vi "Q_learning_get_env_feedback.vi"(8 "A":string, 10 "S":string) -> (0 "R":dbl, 2 "S_":string)   [LabVIEW 2010]
uses:
  Q_learning_Global.vi
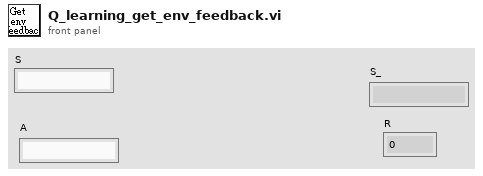
[diagram p1: front panel]
types:
  T1 = cluster{"N_STATES":dbl, "EPSILON":dbl, "ALPHA":dbl, "GAMMA":dbl, "MAX_EPISODES":dbl, "FRESH_TIME":dbl, "ACTIONS":string[]}
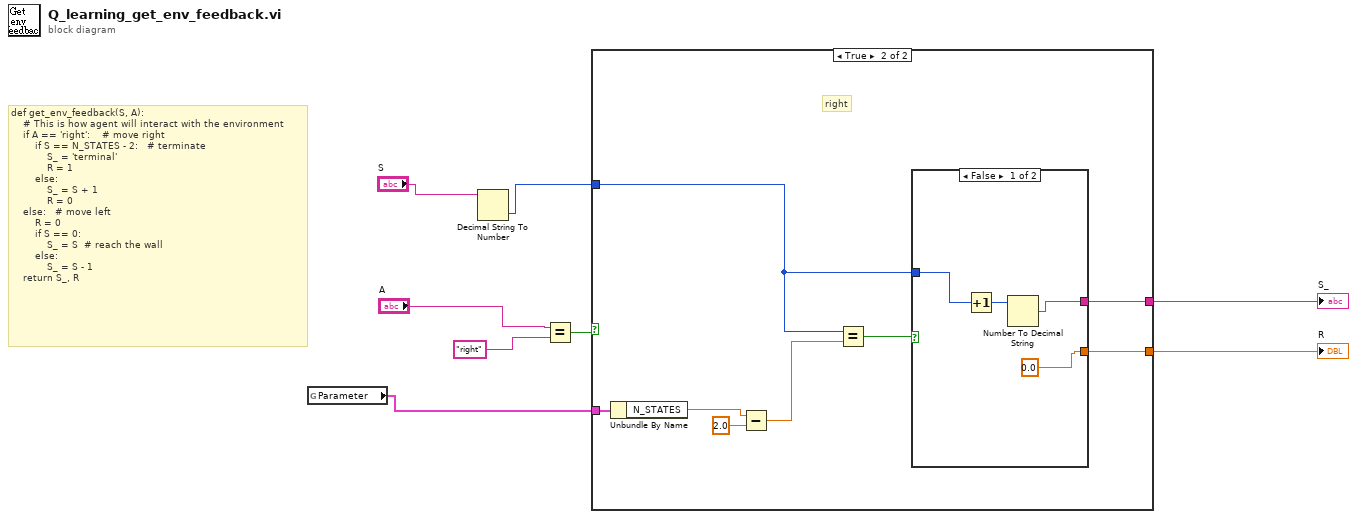
[diagram p0: block diagram]
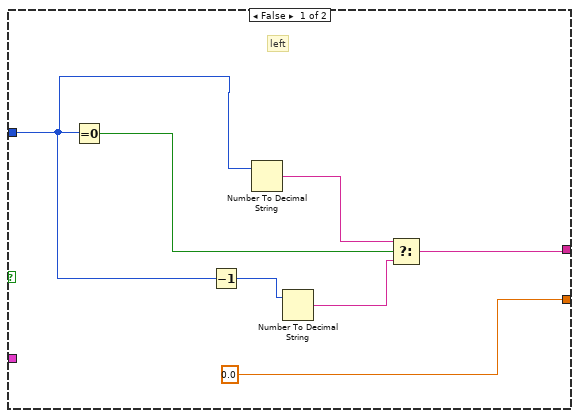
[diagram p2: hidden frame]
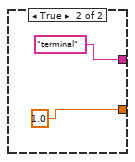
[diagram p3: hidden frame]
diagram:
  # "def get_env_feedback(S, A):\n    # This is how agent will interact with the environment\n    if A == 'right':    # move right\n        if S == N_STATES - 2:   # terminate\n            S_ = 'terminal'\n            R = 1\n        else:\n            S_ = S + 1\n            R = 0\n    else:   # move left\n        R = 0\n        if S == 0:\n            S_ = S  # reach the wall\n        else:\n            S_ = S - 1\n    return S_, R"
  n1 = global read "Q_learning_Global.vi" "Parameter"() -> (w5:T1)
  n2 = Decimal String To Number(string="S") -> (number=w1:i32)  [unwired: 2 in, 1 out]
  n3 = Equal?(x="A", y="right") -> (x = y?=w6:bool)
  n4 = case shown="True" w6 {
    tunnel: w1 -> [w12 w16]
    tunnel: w5 -> [_ w23]
    tunnel: [w9 w18] -> w4
    tunnel: [0.0 ("y") w17] -> w3
    frame False {
      # "left"
      n5 = Equal To 0?(x=w12) -> (x = 0?=w14:bool)
      n6 = Decrement(x=w12) -> (x-1=w11:i32)
      n7 = Number To Decimal String(number=w12) -> (decimal integer string=w13:string)  [unwired: 1 in]
      n8 = Number To Decimal String(number=w11) -> (decimal integer string=w10:string)  [unwired: 1 in]
      n9 = Select(t=w13, s=w14, f=w10) -> (s? t:f=w9:string)
    }
    frame True {
      # "right"
      n10 = Unbundle By Name(w23) -> ("N_STATES"=w22:dbl)
      n11 = Subtract(x=w22, y=2.0) -> (x-y=w20:dbl)
      n12 = Equal?(x=w16, y=w20) -> (x = y?=w19:bool)
      n13 = case shown="False" w19 {
        tunnel: [w25 "terminal"] -> w18
        tunnel: [0.0 ("y") 1.0 ("y")] -> w17
        tunnel: w16 -> [w27 _]
        frame False {
          n14 = Increment(x=w27) -> (x+1=w26:i32)
          n15 = Number To Decimal String(number=w26) -> (decimal integer string=w25:string)  [unwired: 1 in]
        }
        frame True {
        }
      }
    }
  }
  "S_" <- w4
  "R" <- w3
